vi "read xyscan-data.vi"() -> ()   [LabVIEW 2014]
uses:
  <vilib>/Utility/file.llb/Read From Spreadsheet File (DBL).vi
panel:
  out "XY Graph":cluster{dbl[], "all rows":dbl[]}(graph)
  in  "file path (dialog if empty)":path
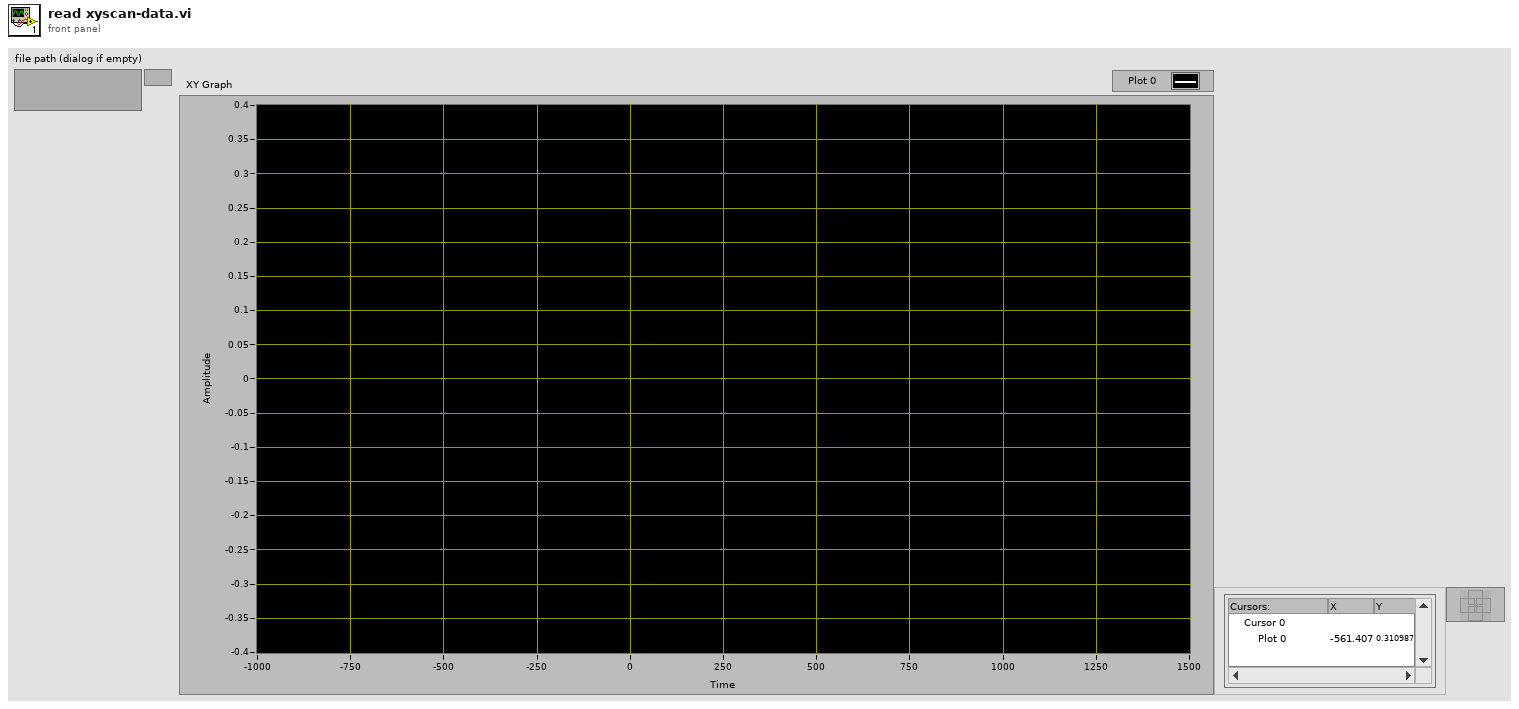
[diagram p1: front panel]
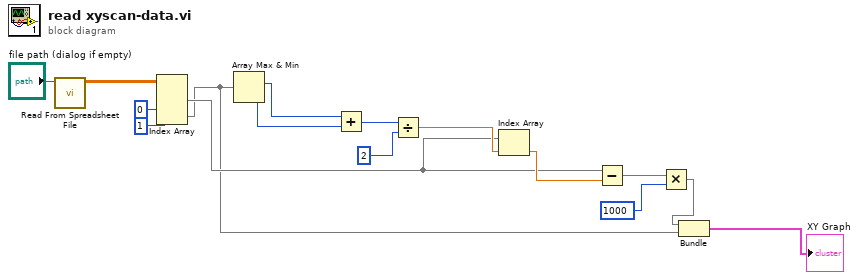
[diagram p0: block diagram]
diagram:
  n1 = call-poly <vilib>:"Read From Spreadsheet File.vi"("file path (dialog if empty)"="file path (dialog if empty)") -> ("all rows"=w15:dbl[][])  [unwired: 6 in, 4 out]
  n2 = Index Array(array=w15, index (col) #1=0 ("disabled index (col)"), index (col) #2=1 ("index (col)")) -> (element #1=w6:dbl[], element #2=w2:dbl[])  [unwired: 2 in]
  n3 = Array Max & Min(array=w2) -> (max index (indices)=w12:i32, min index (indices)=w11:i32)  [unwired: 2 out]
  n4 = Add(x=w12, y=w11) -> (x+y=w10:i32)
  n5 = Divide(x=w10, y=2 ("index (col)")) -> (x/y=w8:dbl)
  n6 = Index Array(array=w6, index=w8) -> (element=w7:dbl)
  n7 = Subtract(x=w6, y=w7) -> (x-y=w5:dbl[])
  n8 = Multiply(x=w5, y=1000 ("index (col)")) -> (x*y=w3:dbl[])
  n9 = Bundle(w3, "all rows"=w2) -> (→"XY Graph":cluster{dbl[], "all rows":dbl[]})  [unwired: 1 in]
